vi "FGV Modules References.vi"(9 "Module_Refs":T1={"ModuleName"=enum."Controller", "Queue"=refnum, "user event"=refnum, "VI Refnum"=refnum, "ShowFP"=FALSE, "StatesTracking Enabled"=FALSE}, 10 "App Module Ref":refnum<vi>, 11 "FGV Ref. Function In":T3) -> (0 "error out":errorcluster, 1 "Module_Ref Out":T1={"ModuleName"=enum."Controller", "Queue"=refnum, "user event"=refnum, "VI Refnum"=refnum, "ShowFP"=FALSE, "StatesTracking Enabled"=FALSE}, 3 "All Modules Refs":T1[](array[typedef]))   [LabVIEW 2019, in "Architecture.lvlib"]
doc: "This FGV stores all references from all modules to be used all around the application to access them. \n\nInit: Use it on application startup. \nAdd: Use it once a new module is initialized in the application to store the references of it. \nGet: Pass a module name to search its references and return them on \"Module_Ref Out\" output. \nGet All: returns all references on \"All modules refs.\"\nDispose: Use it to close all references for all modules. To be used on application stop sequence."
uses:
  Architecture.lvlib
  Typedefs/FGV Ref. Modules Function.ctl
  Typedefs/Module References.ctl
  Typedefs/Enum_Module_Name.ctl
  Typedefs/Message.ctl
panel:
  in  "error in":errorcluster
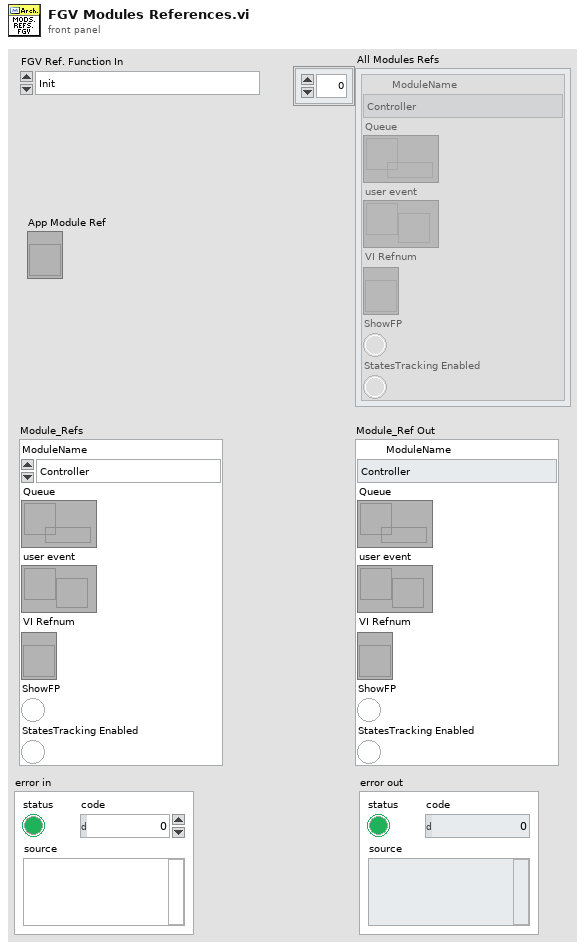
[diagram p1: front panel]
types:
  T1 = typedef "Architecture.lvlib/Module References.ctl" = cluster{"ModuleName":T2, "Queue":refnum<queue>, "user event":refnum<user-event>, "VI Refnum":refnum<vi>, "ShowFP":bool, "StatesTracking Enabled":bool}
  T2 = typedef "Architecture.lvlib/Enum_Module_Name.ctl" = enum16{"Configuration", "Error_Handler", "Log", "Database", "Controller", "User Console", "Display Console", "Sensor Interface"}
  T3 = typedef "Architecture.lvlib/FGV Ref. Modules Function.ctl" = enum16{"Init ", "Add Module", "Get Module", "Get All", "Add Asynchronous Run Ref", "Dispose"}
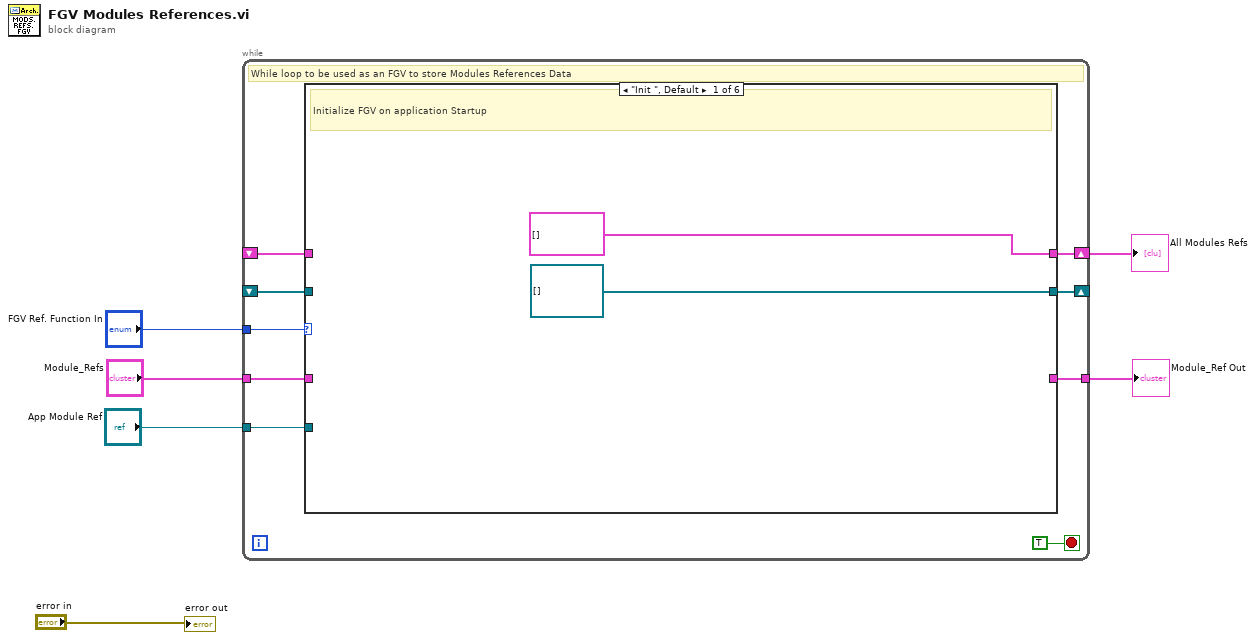
[diagram p0: block diagram]
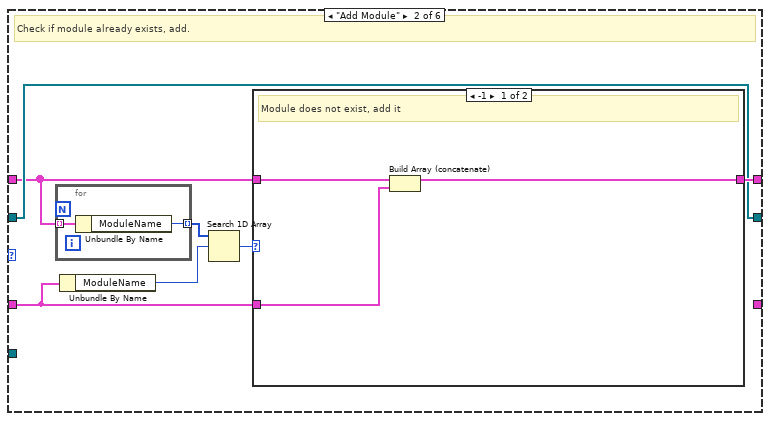
[diagram p2: hidden frame]
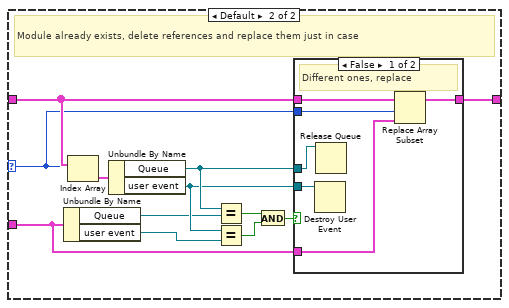
[diagram p3: hidden frame]
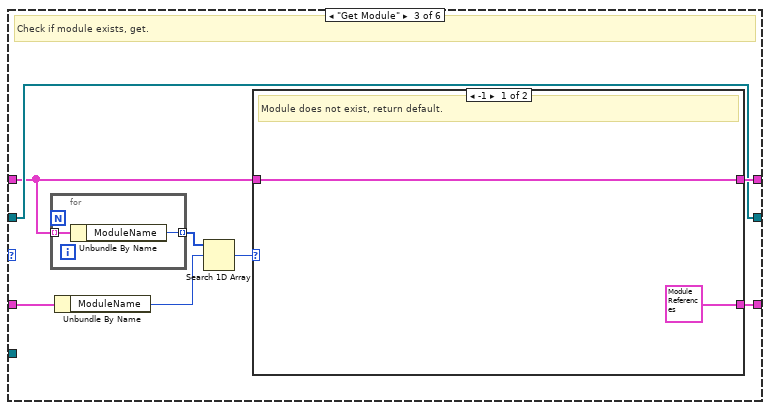
[diagram p5: hidden frame]
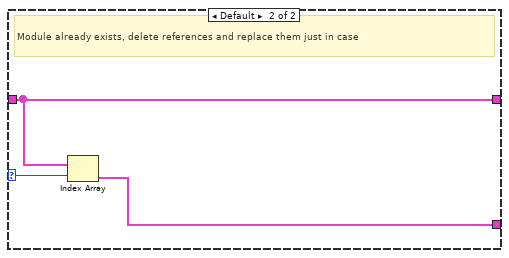
[diagram p6: hidden frame]
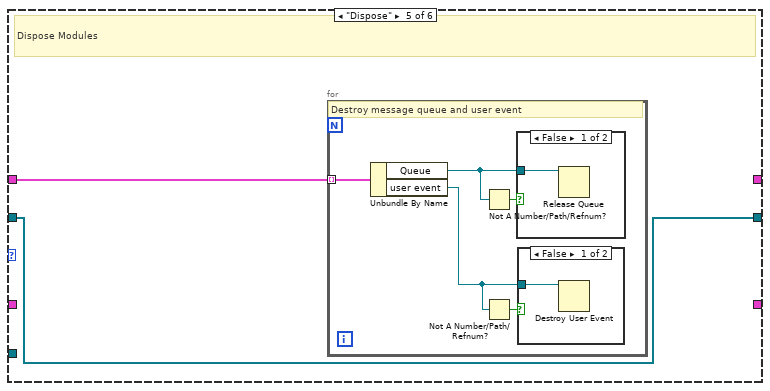
[diagram p8: hidden frame]
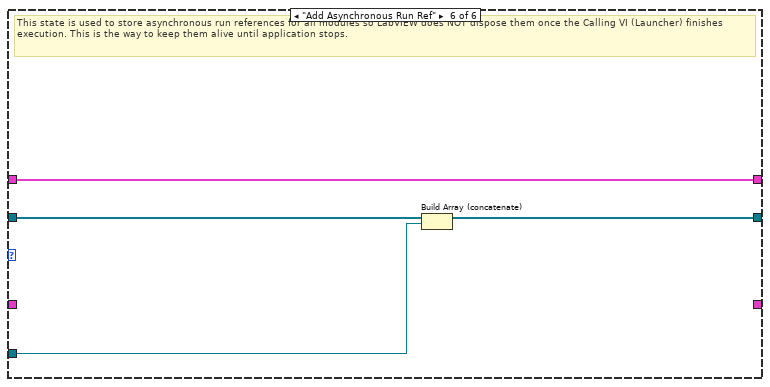
[diagram p11: hidden frame]
diagram:
  n1 = while {
    tunnel: "FGV Ref. Function In" -> [w14]
    shift-right: [w13] -> w3
    shift-left: _ -> [w12]
    tunnel: "Module_Refs" -> [w11]
    tunnel: [w10] -> w4
    tunnel: "App Module Ref" -> [w9]
    shift-right: [w8] -> _
    shift-left: _ -> [w7]
    stop <- TRUE stop-if-true
    # "While loop to be used as an FGV to store Modules References Data"
    n2 = case shown="\"Init \", Default" w14 {
      tunnel: [T1[] [] w24 w55 w65 _ w75] -> w13
      tunnel: w12 -> [_ w19 w50 w65 w67 w75]
      tunnel: w11 -> [_ w21 w54 _ _ _]
      tunnel: [_ _ w53 _ _ _] -> w10
      tunnel: w9 -> [_ _ _ _ _ w76]
      tunnel: [refnum<vi>[] [] ("App Module Ref") w23 w52 w64 w66 w77] -> w8
      tunnel: w7 -> [_ w23 w52 w64 w66 w78]
      frame "Init ", Default {
        # "Initialize FGV on application Startup"
      }
      frame "Add Module" {
        # "Check if module already exists, add."
        n3 = for {
          tunnel: w19 -> [w26] mode=indexing
          tunnel: [w25] -> w22 mode=indexing
          n4 = Unbundle By Name(w26) -> ("ModuleName"=w25:T2)
        }
        n5 = Unbundle By Name(w21) -> ("ModuleName"=w20:T2)
        n6 = Search 1D Array(1D array=w22, element=w20) -> (index of element=w18:i32)  [unwired: 1 in]
        n7 = case shown="-1" w18 {
          selector: w18 -> [_ w31]
          tunnel: w19 -> [w29 w41]
          tunnel: [w28 w39] -> w24
          tunnel: w21 -> [w27 w30]
          frame -1 {
            # "Module does not exist, add it"
            n8 = Build Array (concatenate)(w29, w27) -> (w28:T1[])
          }
          frame Default {
            # "Module already exists, delete references and replace them just in case"
            n9 = Unbundle By Name(w30) -> ("Queue"=w36:refnum<queue>, "user event"=w35:refnum<user-event>)
            n10 = Index Array(array=w41, index=w31) -> (element=w40:T1)
            n11 = Unbundle By Name(w40) -> ("Queue"=w38:refnum<queue>, "user event"=w37:refnum<user-event>)
            n12 = Equal?(x=w38, y=w36) -> (x = y?=w34:bool)
            n13 = Equal?(x=w37, y=w35) -> (x = y?=w33:bool)
            n14 = And(x=w34, y=w33) -> (x .and. y?=w32:bool)
            n15 = case shown="False" w32 {
              tunnel: w41 -> [w47 w48]
              tunnel: [w46 w48] -> w39
              tunnel: w38 -> [w45 _]
              tunnel: w37 -> [w44 _]
              tunnel: w31 -> [w43 _]
              tunnel: w30 -> [w42 _]
              frame False {
                # "Different ones, replace"
                n16 = Destroy User Event(user event=w44) -> ()  [unwired: 1 in, 1 out]
                n17 = Release Queue(queue=w45) -> ()  [unwired: 2 in, 3 out]
                n18 = Replace Array Subset(array=w47, new element=w42, index=w43) -> (w46:T1[])
              }
              frame True {
                # "Same refs, do nothing"
              }
            }
          }
        }
      }
      frame "Get Module" {
        # "Check if module exists, get."
        n19 = for {
          tunnel: w50 -> [w58] mode=indexing
          tunnel: [w57] -> w49 mode=indexing
          n20 = Unbundle By Name(w58) -> ("ModuleName"=w57:T2)
        }
        n21 = Unbundle By Name(w54) -> ("ModuleName"=w51:T2)
        n22 = Search 1D Array(1D array=w49, element=w51) -> (index of element=w56:i32)  [unwired: 1 in]
        n23 = case shown="-1" w56 {
          selector: w56 -> [_ w62]
          tunnel: w50 -> [w60 w63]
          tunnel: [w60 w63] -> w55
          tunnel: [T1 {"ModuleName"=enum."Controller", "Queue"=refnum, "user event"=refnum, "VI Refnum"=refnum, "ShowFP"=FALSE, "StatesTracking Enabled"=FALSE} ("Module_Ref Out") w61] -> w53
          frame -1 {
            # "Module does not exist, return default."
          }
          frame Default {
            # "Module already exists, delete references and replace them just in case"
            n24 = Index Array(array=w63, index=w62) -> (element=w61:T1)
          }
        }
      }
      frame "Get All" {
        # "Return all modules"
      }
      frame "Dispose" {
        # "Dispose Modules"
        n25 = for {
          tunnel: w67 -> [w72] mode=indexing
          # "Destroy message queue and user event"
          n26 = Unbundle By Name(w72) -> ("Queue"=w71:refnum<queue>, "user event"=w69:refnum<user-event>)
          n27 = Not A Number/Path/Refnum?(number/path/refnum=w71) -> (NaN/Path/Refnum?=w70:bool)
          n28 = Not A Number/Path/Refnum?(number/path/refnum=w69) -> (NaN/Path/Refnum?=w68:bool)
          n29 = case shown="False" w70 {
            tunnel: w71 -> [w74 _]
            frame False {
              n30 = Release Queue(queue=w74) -> ()  [unwired: 2 in, 3 out]
            }
            frame True {
            }
          }
          n31 = case shown="False" w68 {
            tunnel: w69 -> [w73 _]
            frame False {
              n32 = Destroy User Event(user event=w73) -> ()  [unwired: 1 in, 1 out]
            }
            frame True {
            }
          }
        }
      }
      frame "Add Asynchronous Run Ref" {
        # "This state is used to store asynchronous run references for all modules so LabVIEW does NOT dispose them once the Calling VI (Launcher) finishes execution. This is the way to keep them alive until application stops."
        n33 = Build Array (concatenate)(w78, w76) -> (w77:refnum<vi>[])
      }
    }
  }
  "Module_Ref Out" <- w4
  "All Modules Refs" <- w3
  "error out" <- "error in"
